vi "Scroll Text Loop.vi"(10 "Output Ref":refnum<vi>, 11 "Exit Ref":refnum<vi>) -> ()   [LabVIEW 2018]
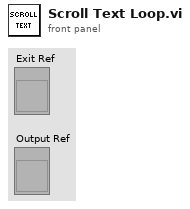
[diagram p1: front panel]
types:
  T1 = typedef "Output Indicator.ctl" = string
  T2 = typedef "Exit Control.ctl" = bool
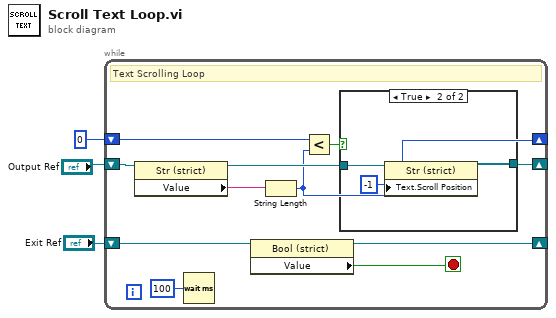
[diagram p0: block diagram]
diagram:
  n1 = while {
    shift-right: [w6] -> _
    shift-left: 0 ("Numeric") -> [w10]
    shift-right: [w7] -> _
    shift-left: "Output Ref" -> [w12]
    shift-right: [w4] -> _
    shift-left: "Exit Ref" -> [w5]
    stop <- w14 stop-if-true
    # "Text Scrolling Loop"
    n2 = property class="Str (strict)"(reference=w12) -> (reference out=w8:refnum<vi>, "Value"=w11:T1)  [unwired: 1 in, 1 out]
    n3 = Wait (ms)(milliseconds to wait=u32 100) -> ()  [unwired: 1 out]
    n4 = property class="Bool (strict)"(reference=w5) -> (reference out=w4:refnum<vi>, "Value"=w14:T2)  [unwired: 1 in, 1 out]
    n5 = String Length(string=w11) -> (length=w6:i32)
    n6 = Less?(x=w10, y=w6) -> (x < y?=w9:bool)
    n7 = case shown="True" w9 {
      tunnel: w8 -> [w15 w17]
      tunnel: [w15 w16] -> w7
      frame False {
      }
      frame True {
        n8 = property class="Str (strict)"(reference=w17, "Text.Scroll Position"=-1) -> (reference out=w16:refnum<vi>)  [unwired: 1 in, 1 out]
      }
    }
  }
